vi "Method Tree Tag to FQN.vi"(3 "Method Tree Tag":string) -> (0 "Message Type":T1, 1 "Method FQN":string)   [LabVIEW 2023, in "Message Maker.lvclass"]
uses:
  Message Maker.lvclass
  Message Type.ctl
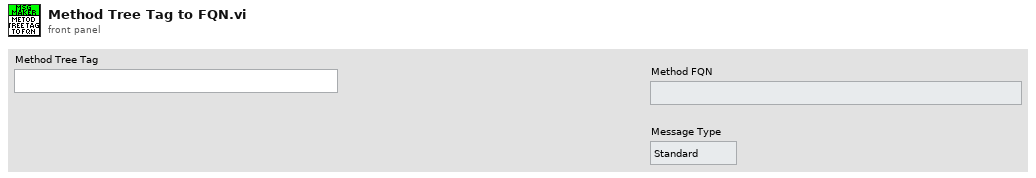
[diagram p1: front panel]
types:
  T1 = typedef "Message Maker.lvclass/Message Type.ctl" = enum16{"Standard", "Async"}
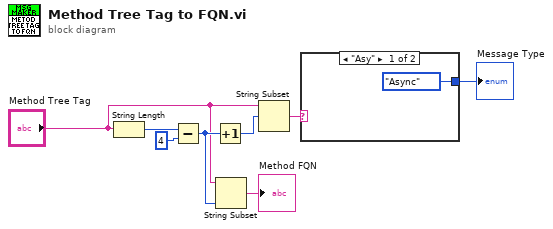
[diagram p0: block diagram]
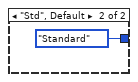
[diagram p2: hidden frame]
diagram:
  n1 = String Length(string="Method Tree Tag") -> (length=w8:i32)
  n2 = Subtract(x=w8, y=4) -> (x-y=w5:i32)
  n3 = Increment(x=w5) -> (x+1=w3:i32)
  n4 = String Subset(string="Method Tree Tag", length (rest)=w5) -> (substring=→"Method FQN":string)  [unwired: 1 in]
  n5 = String Subset(string="Method Tree Tag", offset (0)=w3) -> (substring=w2:string)  [unwired: 1 in]
  n6 = case shown="\"Asy\"" w2 {
    tunnel: [Message_Type."Async" ("Message Type") Message_Type."Standard" ("Message Type")] -> w1
    frame "Asy" {
    }
    frame "Std", Default {
    }
  }
  "Message Type" <- w1
